vi "request_to_server.vi"() -> ()   [LabVIEW 2023]
uses:
  <vilib>/addons/_JKI.lib/REST Client/classes/REST Client/REST Client.lvclass
  System.Windows.Forms
panel:
  in  "load_from_file":bool
  in  "acquisition_from_arduino":bool
  in  "stop_button":bool
  in  "help_button":bool
  out "?":string
  in  "?":u16(ring) items=["Minimum Humidity", "Maximum Humidity", "Average Humidity", "Minimum Temperature", "Maximum Temperature", "Average Temperature", ""]
  in  "Seleziona una data":refnum<k24>(container)
  in  "OK Button":bool
  # "REQUEST TO SERVER"
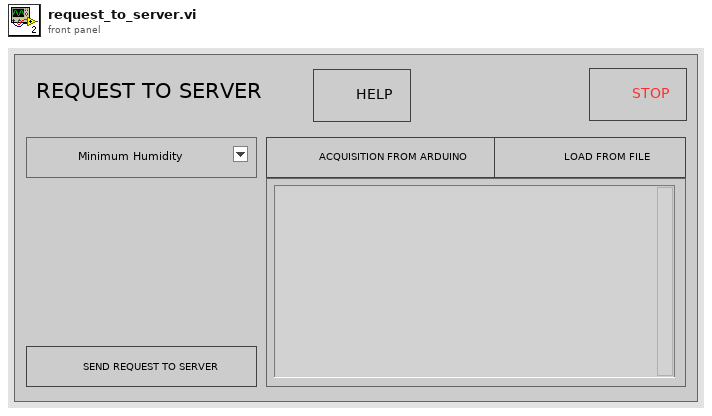
[diagram p1: front panel]
types:
  T1 = enum32{"Invalid", "Standard", "Closed", "Hidden", "Minimized", "Maximized"}
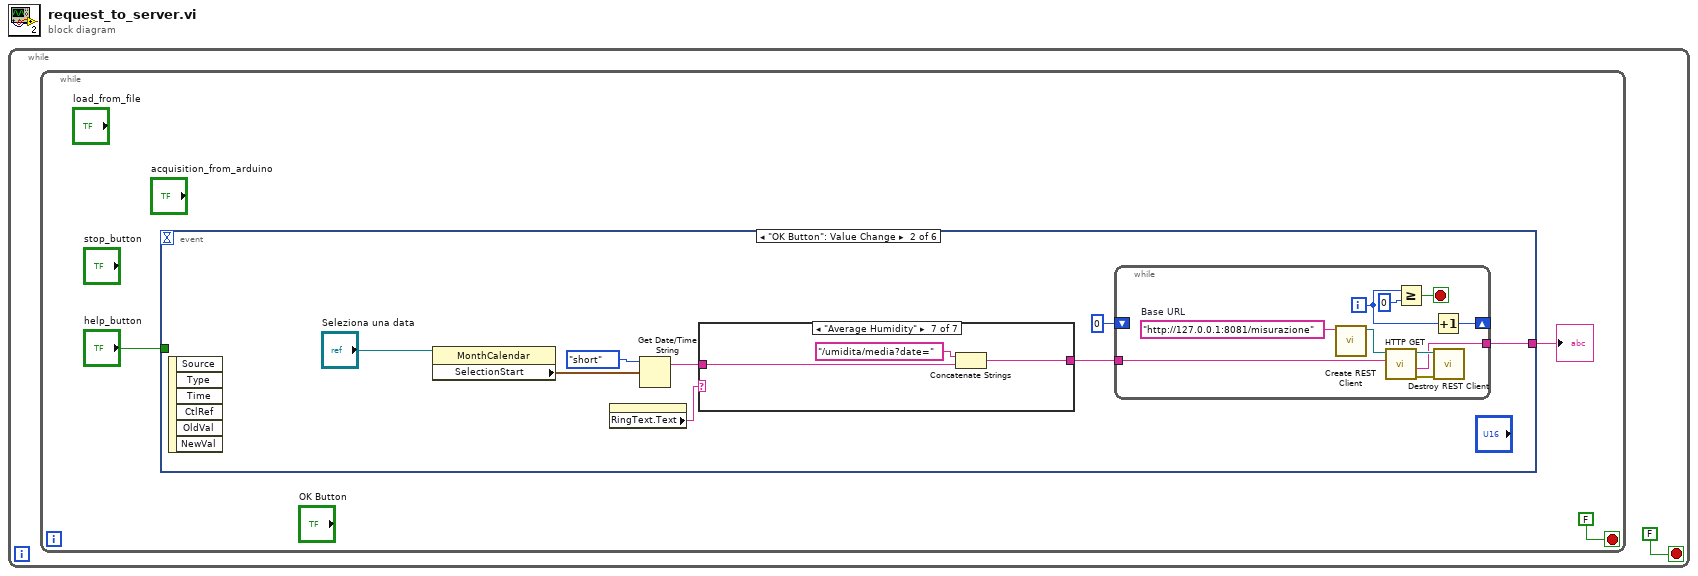
[diagram p0: block diagram]
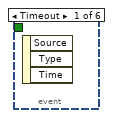
[diagram p2: hidden frame]
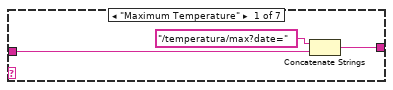
[diagram p3: hidden frame]
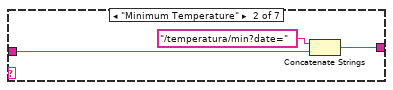
[diagram p4: hidden frame]
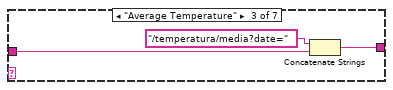
[diagram p5: hidden frame]
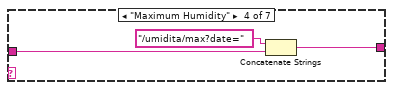
[diagram p6: hidden frame]
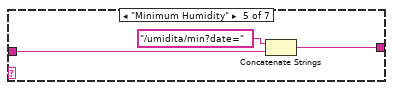
[diagram p7: hidden frame]
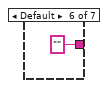
[diagram p8: hidden frame]
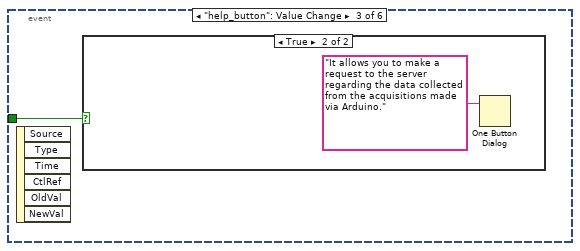
[diagram p9: hidden frame]
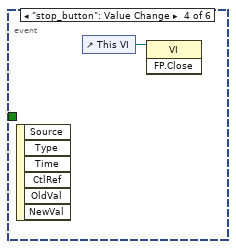
[diagram p11: hidden frame]
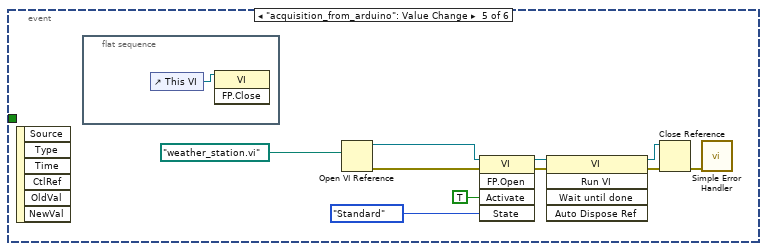
[diagram p12: hidden frame]
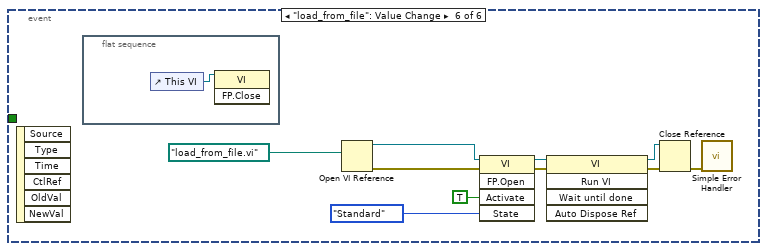
[diagram p13: hidden frame]
diagram:
  n1 = while {
    stop <- FALSE stop-if-true
    n2 = while {
      stop <- FALSE stop-if-true
      n3 = event shown="[1] \"OK Button\": Value Change" {
        selector: _ -> [_ _ _ _ _ _]
        dyn-events: _ -> [_ _ _ _ _ _]
        timeout: _ -> [_ _ _ _ _ _]
        tunnel: [_ w11 _ _ _ _] -> w3
        tunnel: "help_button" -> [_ _ w42 _ _ _]
        event Timeout {
          n4 = event-data() -> ()  [unwired: 1 in, 3 out]
        }
        event "OK Button": Value Change {
          n5 = event-data() -> ()  [unwired: 1 in, 6 out]
          n6 = property class="MonthCalendar"(reference="Seleziona una data") -> ("SelectionStart"=w8:timestamp)  [unwired: 1 in, 2 out]
          n7 = property class="Ring (strict)"() -> ("RingText.Text"=w10:string)  [unwired: 2 in, 2 out]
          n8 = Get Date/Time String(date format (0)=enum16{"short", "long", "abbreviated"}."short", seconds (now)=w8) -> (date string=w9:string)  [unwired: 1 in, 1 out]
          n9 = case shown="\"Average Humidity\"" w10 {
            tunnel: w9 -> [w14 w17 w20 w23 w25 _ w30]
            tunnel: [w13 w16 w19 w22 w26 "" w29] -> w6
            frame "Maximum Temperature" {
              n10 = Concatenate Strings("/temperatura/max?date=" ("Path"), w14) -> (w13:string)
            }
            frame "Minimum Temperature" {
              n11 = Concatenate Strings("/temperatura/min?date=" ("Path"), w17) -> (w16:string)
            }
            frame "Average Temperature" {
              n12 = Concatenate Strings("/temperatura/media?date=" ("Path"), w20) -> (w19:string)
            }
            frame "Maximum Humidity" {
              n13 = Concatenate Strings("/umidita/max?date=" ("Path"), w23) -> (w22:string)
            }
            frame "Minimum Humidity" {
              n14 = Concatenate Strings("/umidita/min?date=" ("Path"), w25) -> (w26:string)
            }
            frame Default {
            }
            frame "Average Humidity" {
              n15 = Concatenate Strings("/umidita/media?date=" ("Path"), w30) -> (w29:string)
            }
          }
          n16 = while {
            shift-right: [w39] -> _
            shift-left: 0 -> [_]
            tunnel: w6 -> [w34]
            tunnel: [w32] -> w11
            i -> [w38]
            stop <- w40 stop-if-true
            w33 = "http://127.0.0.1:8081/misurazione"  # Base URL
            n17 = call <vilib>:"Create REST Client.vi"("Base URL"=w33) -> ("REST Client out"=w35:refnum<class "REST Client.lvclass">)  [unwired: 9 in, 1 out]
            n18 = call-dynamic "HTTP GET.vi"("Path"=w34, "REST Client in"=w35) -> ("error out"=w37:errorcluster, "Response body"=w32:string, "REST Client out"=w36:refnum<class "REST Client.lvclass">)  [unwired: 4 in, 3 out]
            n19 = Greater Or Equal?(x=w38, y=0) -> (x >= y?=w40:bool)
            n20 = Increment(x=w38) -> (x+1=w39:i32)
            n21 = call-dynamic "Destroy REST Client.vi"("error in (no error)"=w37, "REST Client in"=w36) -> ()  [unwired: 9 in, 1 out]
          }
        }
        event "help_button": Value Change {
          n22 = event-data() -> ()  [unwired: 1 in, 6 out]
          n23 = case shown="True" w42 {
            frame False {
            }
            frame True {
              n24 = One Button Dialog(message="It allows you to make a request to the server regarding the data collected from the acquisitions made via Arduino.") -> ()  [unwired: 1 in, 1 out]
            }
          }
        }
        event "stop_button": Value Change {
          n25 = event-data() -> ()  [unwired: 1 in, 6 out]
          n26 = control-ref of="This VI"() -> (w44:refnum<vi>)
          n27 = invoke class="VI" method="FP.Close"(reference=w44) -> ()  [unwired: 2 in, 3 out]
        }
        event "acquisition_from_arduino": Value Change {
          n28 = event-data() -> ()  [unwired: 1 in, 6 out]
          n29 = flat-sequence {
            frame #0 {
              n30 = control-ref of="This VI"() -> (w55:refnum<vi>)
              n31 = invoke class="VI" method="FP.Close"(reference=w55) -> ()  [unwired: 2 in, 3 out]
            }
          }
          n32 = Open VI Reference(vi path=path "weather_station.vi") -> (vi reference=w48:refnum<vi>, error out=w49:errorcluster)  [unwired: 5 in]
          n33 = invoke class="VI" method="FP.Open"(reference=w48, error in=w49, "Activate"=TRUE ("Activate?"), "State"=T1."Standard") -> (reference out=w50:refnum<vi>, error out=w51:errorcluster)  [unwired: 1 in, 3 out]
          n34 = invoke class="VI" method="Run VI"(reference=w50, error in=w51) -> (reference out=w53:refnum<vi>, error out=w52:errorcluster)  [unwired: 3 in, 3 out]
          n35 = Close Reference(reference=w53, error in (no error)=w52) -> (error out=w54:errorcluster)
          n36 = call <vilib>:"Simple Error Handler.vi"("error in (no error)"=w54) -> ()  [unwired: 4 in, 5 out]
        }
        event "load_from_file": Value Change {
          n37 = event-data() -> ()  [unwired: 1 in, 6 out]
          n38 = flat-sequence {
            frame #0 {
              n39 = control-ref of="This VI"() -> (w66:refnum<vi>)
              n40 = invoke class="VI" method="FP.Close"(reference=w66) -> ()  [unwired: 2 in, 3 out]
            }
          }
          n41 = Open VI Reference(vi path=path "load_from_file.vi") -> (vi reference=w59:refnum<vi>, error out=w60:errorcluster)  [unwired: 5 in]
          n42 = invoke class="VI" method="FP.Open"(reference=w59, error in=w60, "Activate"=TRUE ("Activate?"), "State"=T1."Standard") -> (reference out=w61:refnum<vi>, error out=w62:errorcluster)  [unwired: 1 in, 3 out]
          n43 = invoke class="VI" method="Run VI"(reference=w61, error in=w62) -> (reference out=w64:refnum<vi>, error out=w63:errorcluster)  [unwired: 3 in, 3 out]
          n44 = Close Reference(reference=w64, error in (no error)=w63) -> (error out=w65:errorcluster)
          n45 = call <vilib>:"Simple Error Handler.vi"("error in (no error)"=w65) -> ()  [unwired: 4 in, 5 out]
        }
      }
      "?" <- w3
    }
  }
